vi "add_header.vi"(8 "error in (no error)":errorcluster, 9 "value":string, 10 "key":string, 11 "Headers in":refnum<class "Headers.lvclass">) -> (0 "error out":errorcluster, 2 "success":bool, 3 "Headers out":refnum<class "Headers.lvclass">)   [LabVIEW 2020, in "reqwest.lvlib" / "Headers.lvclass"]
uses:
  Headers.lvclass
  lv_reqwest_64.dll
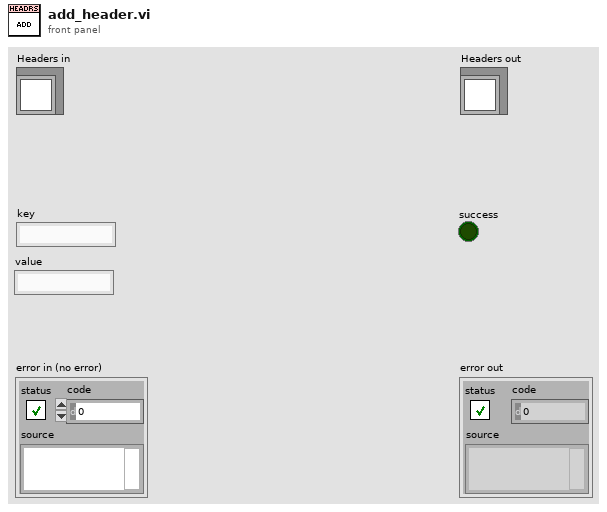
[diagram p1: front panel]
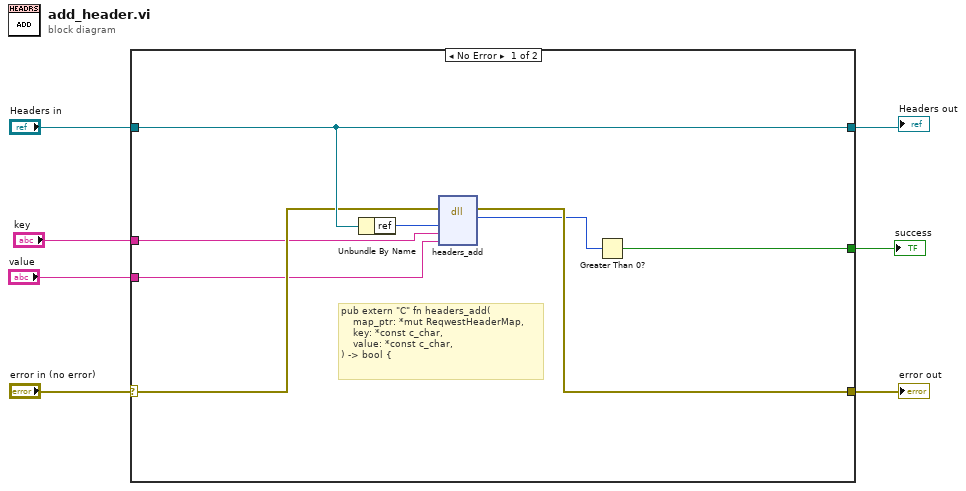
[diagram p0: block diagram]
diagram:
  n1 = case shown="No Error" "error in (no error)" {
    selector: "error in (no error)" -> [w14 w16]
    tunnel: "Headers in" -> [w15 w17]
    tunnel: [w12 w16] -> w4
    tunnel: [w15 w17] -> w5
    tunnel: "key" -> [w13 _]
    tunnel: "value" -> [w10 _]
    tunnel: [w8 _] -> w1
    frame No Error {
      # "pub extern \"C\" fn headers_add(\n    map_ptr: *mut ReqwestHeaderMap,\n    key: *const c_char,\n    value: *const c_char,\n) -> bool {"
      n2 = Unbundle By Name(w15) -> ("ref"=w11:u64)
      n3 = dll-call lib="C:/Projects/reqwest-rs-labview/lv_src/lv_reqwest_*.*" fn="headers_add"(error in=w14, "header_ref"=w11, "key"=w13, "value"=w10) -> (error out=w12:errorcluster, "result"=w9:u8)  [unwired: 5 in, 1 out]
      n4 = Greater Than 0?(x=w9) -> (x > 0?=w8:bool)
    }
    frame Error {
    }
  }
  "error out" <- w4
  "Headers out" <- w5
  "success" <- w1
